vi "List States in Category.vi"(8 "error in (no error)":errorcluster, 10 "Category":string, 11 "JKI SM in":refnum<class "JKI SM.lvclass">) -> (0 "error out":errorcluster, 1 "State Frame Indices":i32[](array[numeric]), 2 "States":string[](array[string]), 3 "JKI SM out":refnum<class "JKI SM.lvclass">, 4 "Category Frame Index":i32)   [LabVIEW 2013, in "JKI State Machine API.lvlib" / "JKI SM.lvclass"]
uses:
  JKI SM.lvclass
  JKI SM.lvclass/JKI SM.ctl
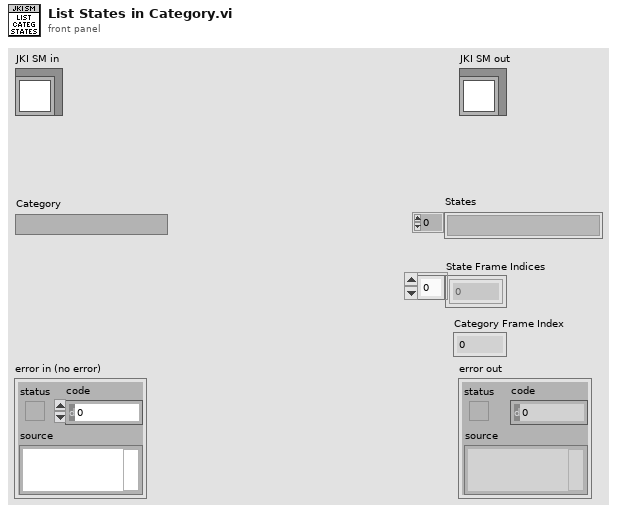
[diagram p1: front panel]
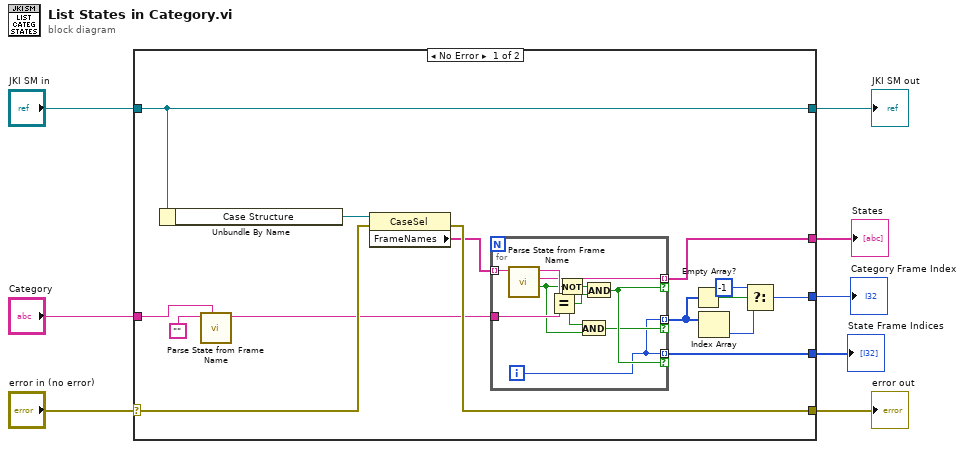
[diagram p0: block diagram]
diagram:
  n1 = case shown="No Error" "error in (no error)" {
    selector: "error in (no error)" -> [w21 w35]
    tunnel: [w20 w35] -> w7
    tunnel: [w23 w34] -> w5
    tunnel: "JKI SM in" -> [w23 w34]
    tunnel: [w18 _] -> w4
    tunnel: "Category" -> [w10 _]
    tunnel: [w17 _] -> w2
    tunnel: [w12 _] -> w1
    frame No Error {
      n2 = Unbundle By Name(w23) -> ("Case Structure"=w22:refnum<vi>)
      n3 = call "Parse State from Frame Name.vi"("Category (Optional)"=w10, "Frame or State Name"="") -> ("Category Name"=w11:string)  [unwired: 5 in, 4 out]
      n4 = property class="CaseSel"(reference=w22, error in=w21) -> (error out=w20:errorcluster, "FrameNames"=w19:string[])  [unwired: 1 out]
      n5 = for {
        tunnel: w11 -> [w31]
        tunnel: w19 -> [w33] mode=indexing
        tunnel: [w30] -> w18 mode=indexing if=w28
        tunnel: [w24] -> w17 mode=indexing if=w28
        tunnel: [w24] -> w16 mode=indexing if=w25
        i -> [w24]
        n6 = call "Parse State from Frame Name.vi"("Frame or State Name"=w33) -> ("is a Category Frame?"=w26:bool, "State Name"=w30:string, "Category Name"=w32:string)  [unwired: 6 in, 2 out]
        n7 = Equal?(x=w32, y=w31) -> (x = y?=w27:bool)
        n8 = Not(x=w26) -> (.not. x?=w29:bool)
        n9 = And(x=w27, y=w26) -> (x .and. y?=w25:bool)
        n10 = And(x=w29, y=w27) -> (x .and. y?=w28:bool)
      }
      n11 = Empty Array?(array=w16) -> (empty?=w15:bool)
      n12 = Index Array(array=w16) -> (element=w14:i32)  [unwired: 1 in]
      n13 = Select(t=-1, s=w15, f=w14) -> (s? t:f=w12:i32)
    }
    frame Error {
    }
  }
  "error out" <- w7
  "JKI SM out" <- w5
  "States" <- w4
  "State Frame Indices" <- w2
  "Category Frame Index" <- w1
